vi "convertClockSourceNames.vi"(8 "error in (no error)":errorcluster, 10 "Clock Source":string, 11 "AnalogOutput in":refnum<class "AnalogOutput.lvclass">) -> (0 "error out":errorcluster, 2 "convertedClockName":string, 3 "AnalogOutput out":refnum<class "AnalogOutput.lvclass">)   [LabVIEW 2011, in "Hardware.lvlib" / "Channels.lvlib" / "AnalogOutput.lvclass"]
uses:
  AnalogOutput.lvclass
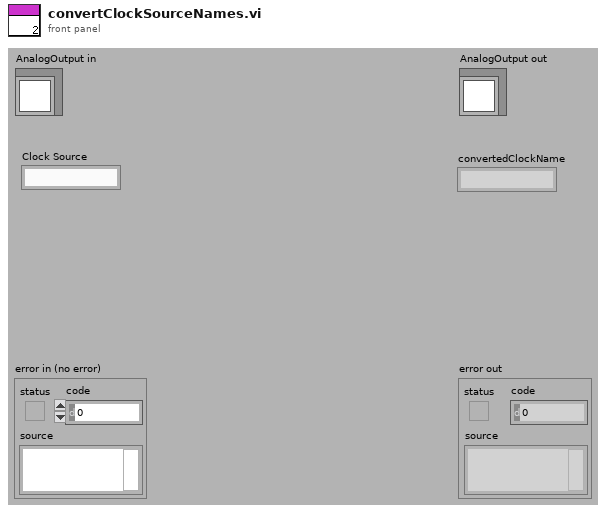
[diagram p1: front panel]
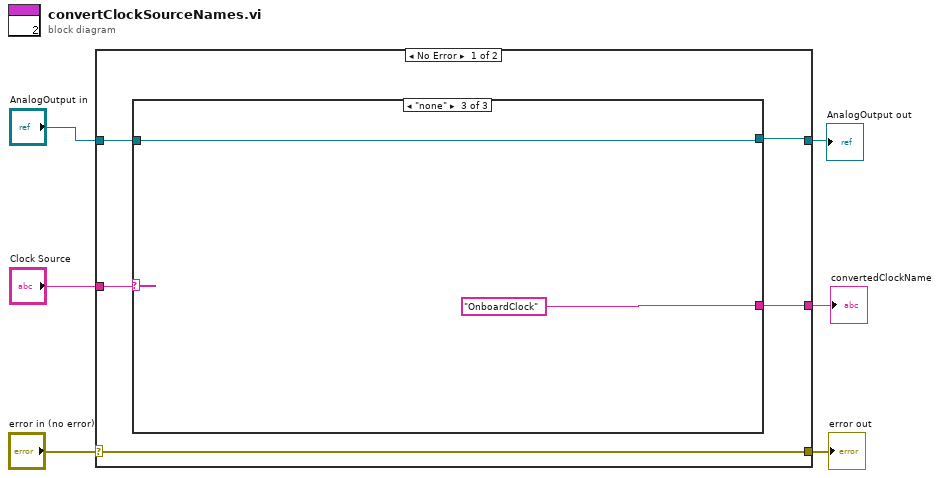
[diagram p0: block diagram]
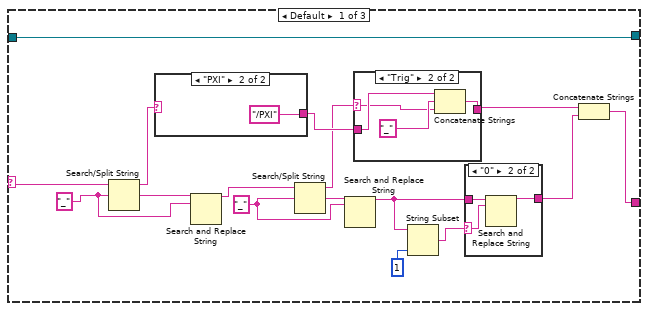
[diagram p2: hidden frame]
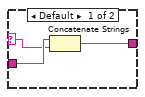
[diagram p4: hidden frame]
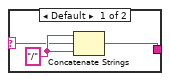
[diagram p5: hidden frame]
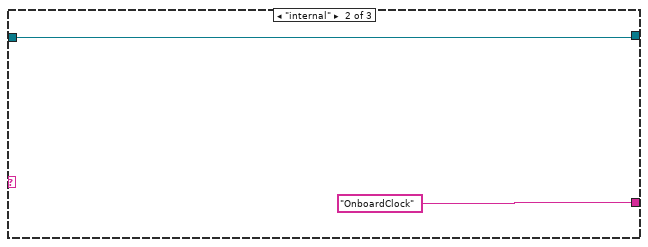
[diagram p6: hidden frame]
diagram:
  n1 = case shown="No Error" "error in (no error)" {
    selector: "error in (no error)" -> [w11 w48]
    tunnel: [w11 w48] -> w5
    tunnel: [w8 w47] -> w3
    tunnel: "AnalogOutput in" -> [w9 w47]
    tunnel: "Clock Source" -> [w10 _]
    tunnel: [w7 _] -> w1
    frame No Error {
      n2 = case shown="\"none\"" w10 {
        selector: w10 -> [w27 _ _]
        tunnel: [w13 "OnboardClock" "OnboardClock"] -> w7
        tunnel: w9 -> [w17 w43 w45]
        tunnel: [w17 w43 w45] -> w8
        frame Default {
          w24 = "_"
          w26 = "_"
          n3 = Search/Split String(string=w27, search string/char (-)=w26) -> (substring before match=w22:string, match + rest of string=w23:string)  [unwired: 1 in, 1 out]
          n4 = case shown="\"PXI\"" w22 {
            selector: w22 -> [w40 _]
            tunnel: [w39 "/PXI"] -> w21
            frame Default {
              w41 = "/"
              n5 = Concatenate Strings(w41, w40, w41) -> (w39:string)
            }
            frame "PXI" {
            }
          }
          n6 = Search and Replace String(input string=w23, search string=w26) -> (result string=w12:string)  [unwired: 6 in, 3 out]
          n7 = Search/Split String(string=w12, search string/char (-)=w24) -> (substring before match=w20:string, match + rest of string=w25:string)  [unwired: 1 in, 1 out]
          n8 = Search and Replace String(input string=w25, search string=w24) -> (result string=w16:string)  [unwired: 6 in, 3 out]
          n9 = case shown="\"Trig\"" w20 {
            selector: w20 -> [w32 w35]
            tunnel: w21 -> [w33 w37]
            tunnel: [w34 w38] -> w15
            frame Default {
              n10 = Concatenate Strings(w33, w32) -> (w34:string)
            }
            frame "Trig" {
              n11 = Concatenate Strings(w37, "_", w35) -> (w38:string)
            }
          }
          n12 = String Subset(string=w16, length (rest)=1) -> (substring=w18:string)  [unwired: 1 in]
          n13 = case shown="\"0\"" w18 {
            selector: w18 -> [_ w30]
            tunnel: w16 -> [w28 w31]
            tunnel: [w28 w29] -> w14
            frame Default {
            }
            frame "0" {
              n14 = Search and Replace String(input string=w31, search string=w30) -> (result string=w29:string)  [unwired: 6 in, 3 out]
            }
          }
          n15 = Concatenate Strings(w15, w14) -> (w13:string)
        }
        frame "internal" {
        }
        frame "none" {
        }
      }
    }
    frame Error {
    }
  }
  "error out" <- w5
  "AnalogOutput out" <- w3
  "convertedClockName" <- w1
